vi "Get Current Turn.vi"(8 "error in (no error)":errorcluster, 11 "Reversi in":refnum<class "Reversi.lvclass">) -> (0 "error out":errorcluster, 2 "Current Turn":T1, 3 "Reversi out":refnum<class "Reversi.lvclass">)   [LabVIEW 2020, in "Reversi.lvlib" / "Reversi.lvclass"]
uses:
  Reversi.lvclass
  Space Ring.ctl
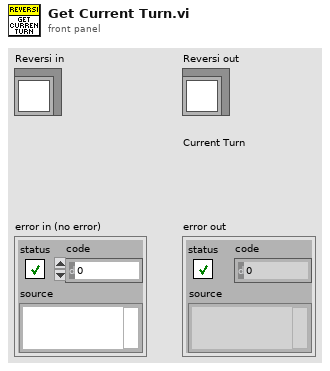
[diagram p1: front panel]
types:
  T1 = typedef "Reversi.lvlib/Reversi.lvclass/Space Ring.ctl" = u16
  T2 = typedef "Reversi.lvlib/Reversi.lvclass/Turn Enum.ctl" = enum16{"Black", "White"}
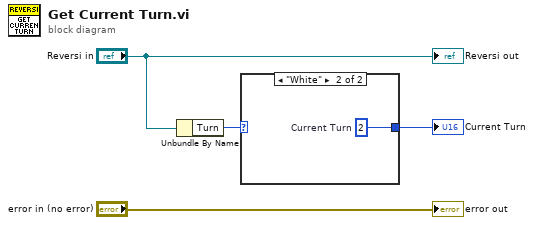
[diagram p0: block diagram]
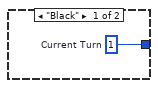
[diagram p2: hidden frame]
diagram:
  n1 = Unbundle By Name("Reversi in") -> ("Turn"=w2:T2)
  n2 = case shown="\"White\"" w2 {
    tunnel: [w5 w6] -> w1
    frame "Black" {
      w5 = T1 1  # Current Turn
    }
    frame "White" {
      w6 = T1 2  # Current Turn
    }
  }
  "Current Turn" <- w1
  "error out" <- "error in (no error)"
  "Reversi out" <- "Reversi in"
